vi "Pin Map Client Create or Update Pin Map.vi"(8 "error in (no error)":errorcluster, 10 "Request Data":T3, 11 "gRPC ID Out":T1) -> (0 "error out":errorcluster, 2 "Response Data":T2, 3 "gRPC ID out":T1)   [LabVIEW 2020]
uses:
  Pin Map Client_lv/Pin Map_client/RPC Messages/ni_measurementlink_pinmap_v1_CreatePinMapFromXmlRequest.ctl
  Pin Map Client_lv/Pin Map_client/RPC Messages/ni_measurementlink_pinmap_v1_PinMap.ctl
  <vilib>/gRPC/LabVIEW gRPC Library/Shared/grpcId.ctl
  Pin Map Client_lv/Pin Map_client/RPC Messages/ni_measurementlink_pinmap_v1_GetPinMapRequest.ctl
  Pin Map Client_lv/Pin Map_client/Pin Map_client.lvlib
  <vilib>/gRPC/LabVIEW gRPC Library/grpc-lvsupport-release.lvlib
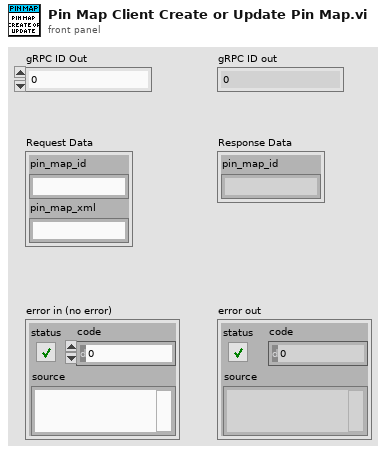
[diagram p1: front panel]
types:
  T1 = typedef "grpc-lvsupport-release.lvlib/grpcId.ctl" = u64
  T2 = typedef "Pin Map_client.lvlib/ni_measurementlink_pinmap_v1_PinMap.ctl" = cluster{"pin_map_id":string}
  T3 = typedef "Pin Map_client.lvlib/ni_measurementlink_pinmap_v1_CreatePinMapFromXmlRequest.ctl" = cluster{"pin_map_id":string, "pin_map_xml":string}
  T4 = typedef "Pin Map_client.lvlib/ni_measurementlink_pinmap_v1_GetPinMapRequest.ctl" = cluster{"pin_map_id":string}
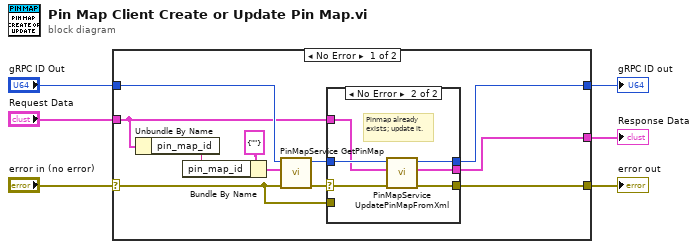
[diagram p0: block diagram]
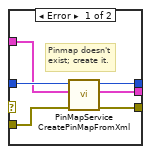
[diagram p2: hidden frame]
diagram:
  n1 = case shown="No Error" "error in (no error)" {
    selector: "error in (no error)" -> [w7 w30]
    tunnel: [w17 _] -> w6
    tunnel: [w16 w30] -> w5
    tunnel: [w15 w31] -> w4
    tunnel: "Request Data" -> [w9 _]
    tunnel: "gRPC ID Out" -> [w14 w31]
    frame No Error {
      n2 = Unbundle By Name(w9) -> ("pin_map_id"=w11:string)
      n3 = Bundle By Name(cluster=T4 {"pin_map_id"=""} ("Request Data"), "pin_map_id"=w11) -> (w10:T4)
      n4 = call "PinMapService GetPinMap.vi"("error in"=w7, "Request Data"=w10, "gRPC ID"=w14) -> ("error out"=w8:errorcluster, "gRPC ID out"=w13:T1)  [unwired: 6 in, 1 out]
      n5 = case shown="No Error" w8 {
        selector: w8 -> [_ w29]
        tunnel: [w23 w25] -> w17
        tunnel: [w22 w26] -> w16
        tunnel: [w21 w24] -> w15
        tunnel: w13 -> [w20 w28]
        tunnel: w9 -> [w19 w27]
        tunnel: w7 -> [w18 _]
        frame Error {
          # "Pinmap doesn't exist; create it."
          n6 = call "PinMapService CreatePinMapFromXml.vi"("error in"=w18, "Request Data"=w19, "gRPC ID"=w20) -> ("error out"=w22:errorcluster, "Response Data"=w23:T2, "gRPC ID out"=w21:T1)  [unwired: 6 in]
        }
        frame No Error {
          # "Pinmap already exists; update it."
          n7 = call "PinMapService UpdatePinMapFromXml.vi"("error in"=w29, "Request Data"=w27, "gRPC ID"=w28) -> ("error out"=w26:errorcluster, "Response Data"=w25:T2, "gRPC ID out"=w24:T1)  [unwired: 6 in]
        }
      }
    }
    frame Error {
    }
  }
  "Response Data" <- w6
  "error out" <- w5
  "gRPC ID out" <- w4
